vi "Init File.vi"(6 "Section":string, 7 "create file if necessary (T)":bool=TRUE, 8 "error in (no error)":errorcluster, 10 "configuration file path":path, 11 "Parameter INI File in":refnum<class "Parameter INI File.lvclass">) -> (0 "error out":errorcluster, 3 "Parameter INI File out":refnum<class "Parameter INI File.lvclass">)   [LabVIEW 2016, in "CD Parameter Manager API.lvlib" / "Parameter INI File.lvclass"]
uses:
  Parameter INI File.lvclass
  <vilib>/Utility/config.llb/NI_LVConfig.lvlib
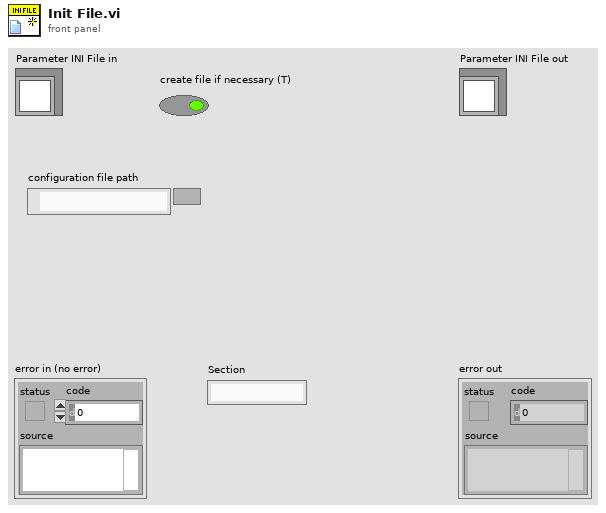
[diagram p1: front panel]
types:
  T1 = typedef "NI_LVConfig.lvlib/Config Data RefNum.ctl" = refnum<k1>
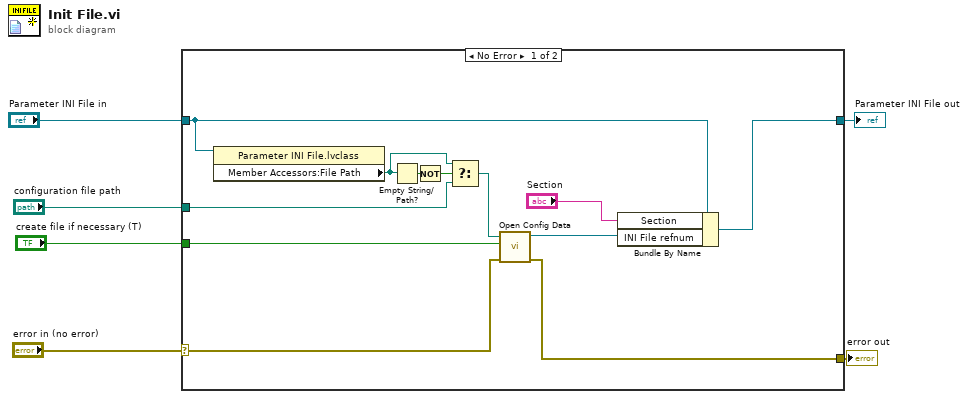
[diagram p0: block diagram]
diagram:
  n1 = case shown="No Error" "error in (no error)" {
    selector: "error in (no error)" -> [w15 w19]
    tunnel: [w18 w20] -> w5
    tunnel: "Parameter INI File in" -> [w7 w20]
    tunnel: "configuration file path" -> [w11 _]
    tunnel: "create file if necessary (T)" -> [w16 _]
    tunnel: [w14 w19] -> w1
    frame No Error {
      n2 = property class="Parameter INI File.lvclass"(reference=w7) -> ("Member Accessors:File Path"=w10:path)  [unwired: 1 in, 2 out]
      n3 = Empty String/Path?(string/path=w10) -> (empty?=w13:bool)
      n4 = Not(x=w13) -> (.not. x?=w12:bool)
      n5 = Select(t=w10, s=w12, f=w11) -> (s? t:f=w9:path)
      n6 = call <vilib>:"Open Config Data.vi"("error in (no error)"=w15, "create file if necessary (T)"=w16, "configuration file path"=w9) -> ("error out"=w14:errorcluster, "refnum"=w17:T1)  [unwired: 6 in, 1 out]
      n7 = Bundle By Name(cluster=w7, "Section"="Section", "INI File refnum"=w17) -> (w18:refnum<class "Parameter INI File.lvclass">)
    }
    frame Error {
    }
  }
  "error out" <- w1
  "Parameter INI File out" <- w5
